vi "Refresh Database Port Compare.vi"(8 "error in":errorcluster, 10 "CAN Cluster":T5, 11 "Port Ref":T8 format="%.0x") -> (0 "error out":errorcluster, 2 "Refresh Port":T1)   [LabVIEW 2020, in "Communication Bus Template System Explorer.lvlib" / "Implementation.lvlib"]
uses:
  Implementation.lvlib
  <vilib>/NI VeriStand/Custom Device API/Custom Device Item Ref.ctl
  Types/Database.ctl
  Types/Frame.ctl
  Types/Signal.ctl
  Types/ECU.ctl
  Types/Refresh Port.ctl
  Types/Refresh Frame.ctl
  Types/Refresh Signal.ctl
  <vilib>/NI VeriStand/Custom Device API/Custom Device Channel Type.ctl
  Scripting/Communication Bus Template Scripting.lvlib
  <vilib>/NI VeriStand/Custom Device API/Custom Device API.lvlib
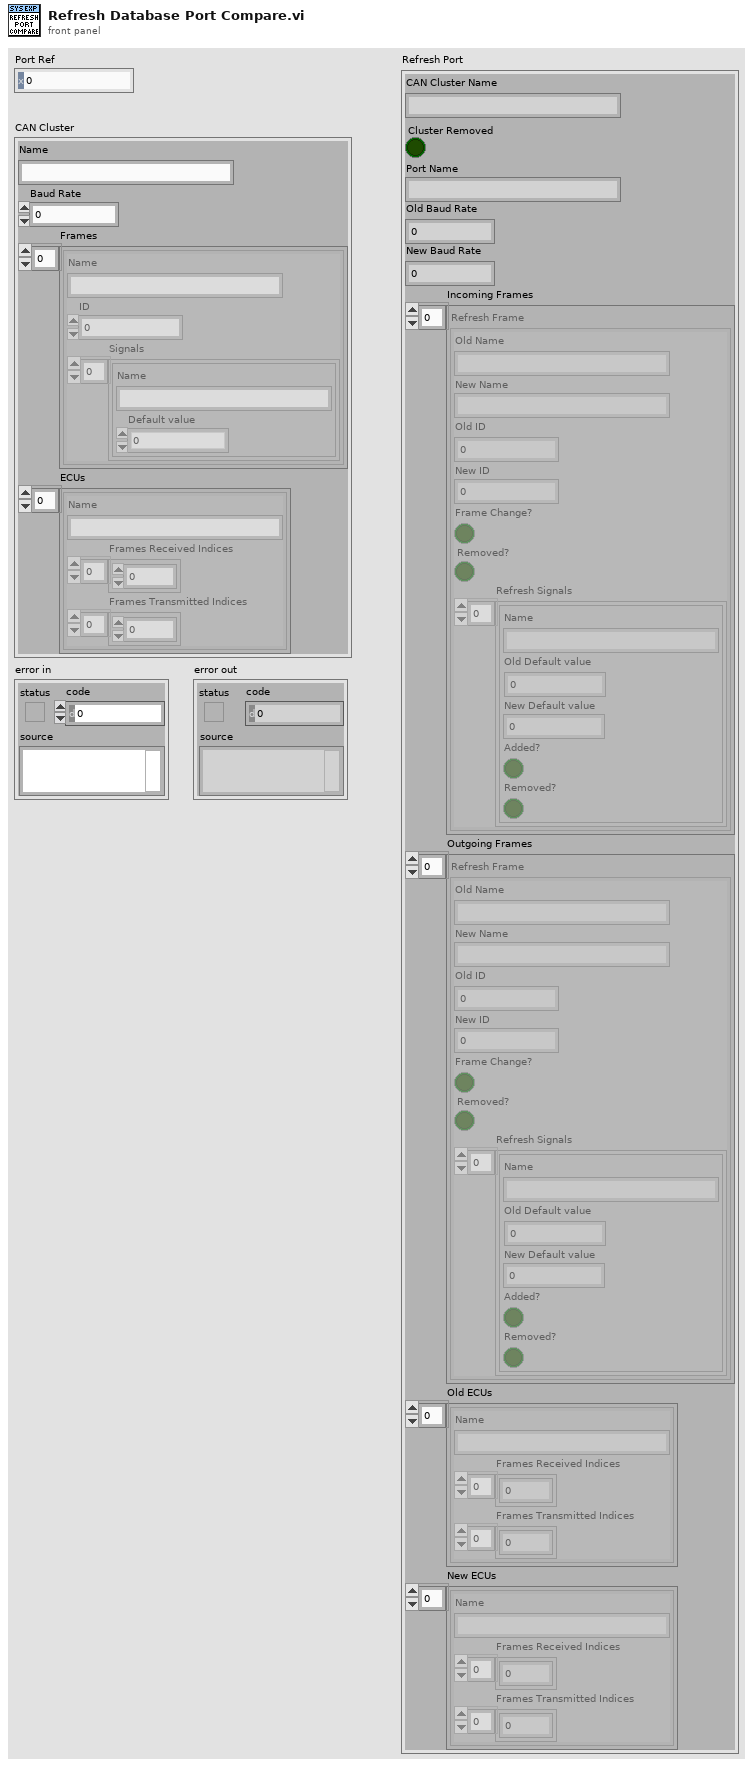
[diagram p1: front panel]
types:
  T1 = typedef "Communication Bus Template System Explorer.lvlib/Implementation.lvlib/Refresh Port.ctl" = cluster{"CAN Cluster Name":string, "Cluster Removed":bool, "Port Name":string, "Old Baud Rate":u64, "New Baud Rate":u64, "Incoming Frames":T2[], "Outgoing Frames":T2[], "Old ECUs":T4[], "New ECUs":T4[]}
  T2 = typedef "Communication Bus Template System Explorer.lvlib/Implementation.lvlib/Refresh Frame.ctl" = cluster{"Old Name":string, "New Name":string, "Old ID":u32, "New ID":u32, "Frame Change?":bool, "Removed?":bool, "Refresh Signals":T3[]}
  T3 = typedef "Communication Bus Template System Explorer.lvlib/Implementation.lvlib/Refresh Signal.ctl" = cluster{"Name":string, "Old Default value":dbl, "New Default value":dbl, "Added?":bool, "Removed?":bool}
  T4 = typedef "Communication Bus Template System Explorer.lvlib/Implementation.lvlib/ECU.ctl" = cluster{"Name":string, "Frames Received Indices":u32[], "Frames Transmitted Indices":u32[]}
  T5 = typedef "Communication Bus Template System Explorer.lvlib/Implementation.lvlib/Database.ctl" = cluster{"Name":string, "Baud Rate":u64, "Frames":T6[], "ECUs":T4[]}
  T6 = typedef "Communication Bus Template System Explorer.lvlib/Implementation.lvlib/Frame.ctl" = cluster{"Name":string, "ID":u32, "Signals":T7[]}
  T7 = typedef "Communication Bus Template System Explorer.lvlib/Implementation.lvlib/Signal.ctl" = cluster{"Name":string, "Default value":dbl}
  T8 = typedef "Custom Device API.lvlib/Custom Device Item Ref.ctl" = u64
  T9 = typedef "Custom Device API.lvlib/Custom Device Channel Type.ctl" = enum16{"Input", "Output"}
  T10 = typedef "Custom Device API.lvlib/Custom Device Channel.ctl" = cluster{"Type":T9, "Units":string, "Default Value":dbl, "Faultable":bool, "Scalable":bool}
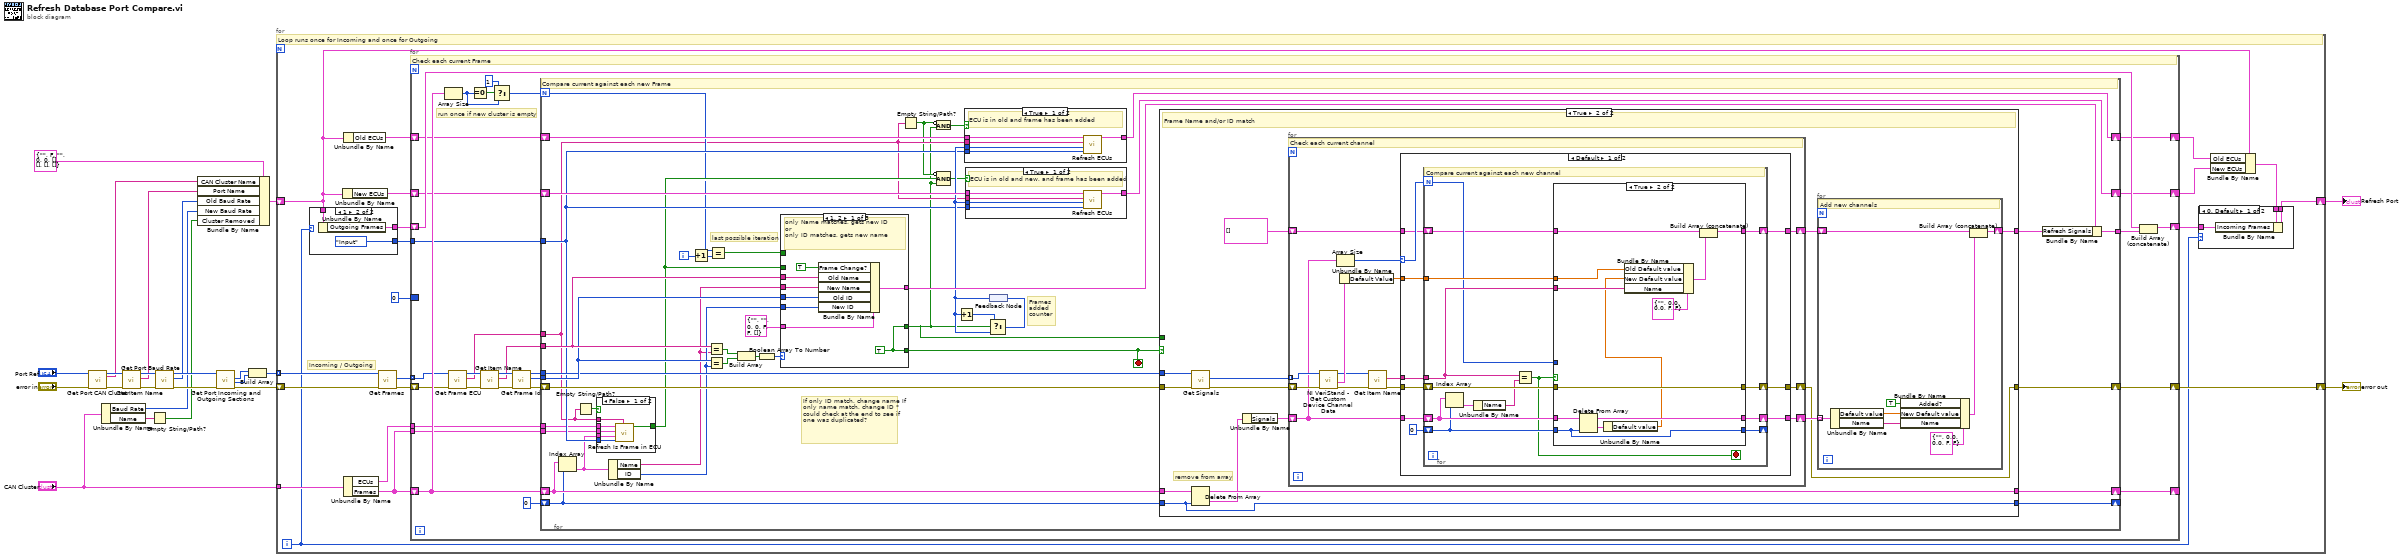
[diagram p0: block diagram]
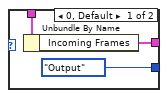
[diagram p2: hidden frame]
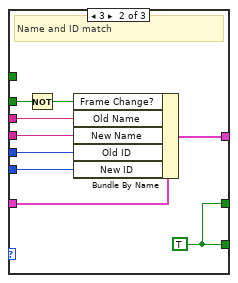
[diagram p6: hidden frame]
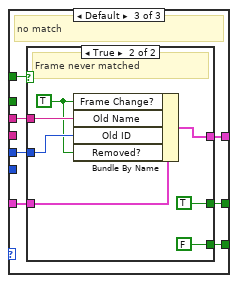
[diagram p7: hidden frame]
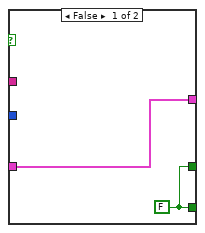
[diagram p8: hidden frame]
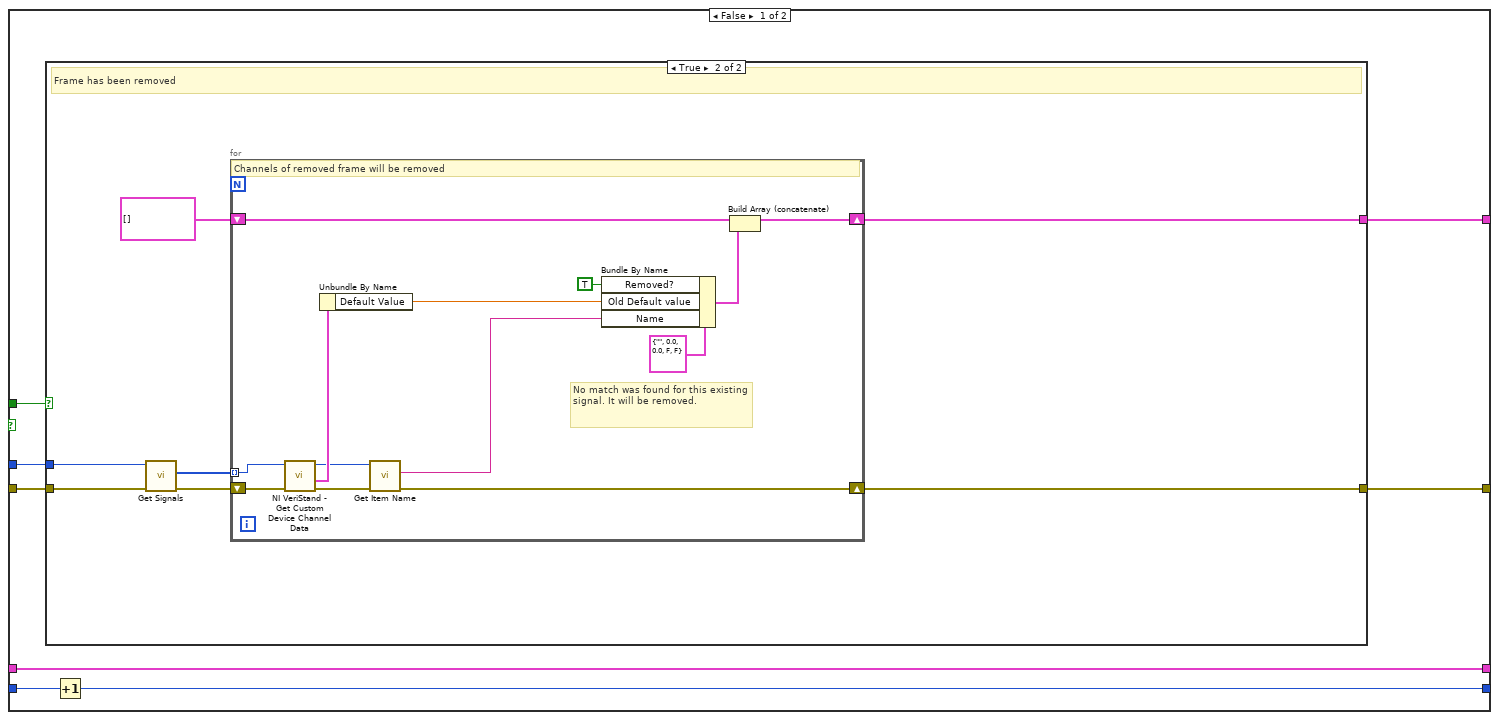
[diagram p9: hidden frame]
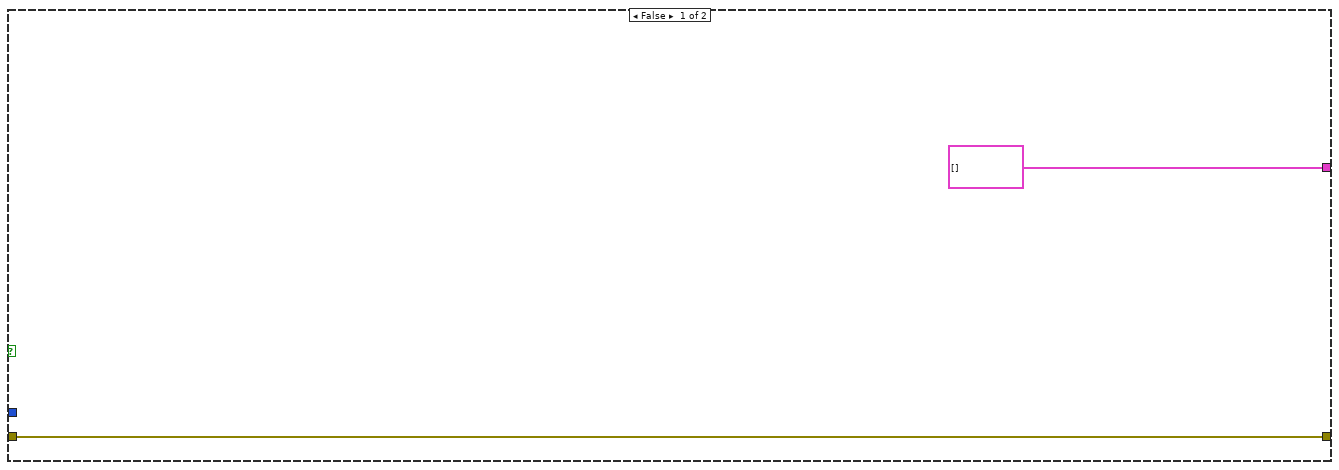
[diagram p10: hidden frame]
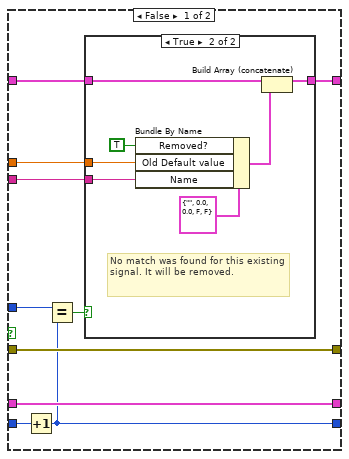
[diagram p11: hidden frame]
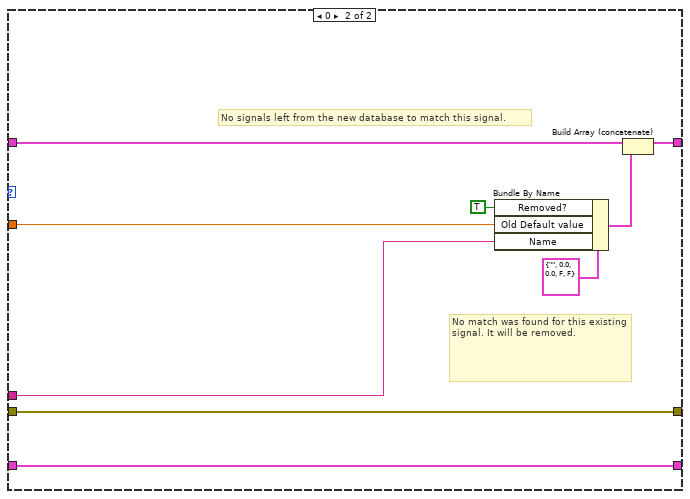
[diagram p13: hidden frame]
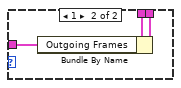
[diagram p14: hidden frame]
diagram:
  n1 = call "Get Port CAN Cluster.vi"("error in"="error in", "Port Ref"="Port Ref") -> ("error out"=w4:errorcluster, "CAN Cluster"=w3:string, "Port Ref out"=w6:T8)  [unwired: 7 in]
  n2 = Unbundle By Name("CAN Cluster") -> ("Baud Rate"=w10:u64, "Name"=w2:string)
  n3 = call "Get Item Name.vi"("error in"=w4, "Item Ref"=w6) -> ("error out"=w15:errorcluster, "Name"=w12:string, "Item Ref out"=w14:T8)  [unwired: 7 in]
  n4 = Empty String/Path?(string/path=w2) -> (empty?=w1:bool)
  n5 = call "Get Port Baud Rate.vi"("error in"=w15, "Port Ref"=w14) -> ("error out"=w22:errorcluster, "Baud Rate"=w11:u32, "Port Ref out"=w23:T8)  [unwired: 7 in]
  n6 = Bundle By Name(cluster=T1 {"CAN Cluster Name"="", "Cluster Removed"=FALSE, "Port Name"="", "Old Baud Rate"=0, "New Baud Rate"=0, "Incoming Frames"=[], "Outgoing Frames"=[], "Old ECUs"=[], "New ECUs"=[]} ("Refresh Port"), "CAN Cluster Name"=w3, "Port Name"=w12, "Old Baud Rate"=w11, "New Baud Rate"=w10, "Cluster Removed"=w1) -> (w9:T1)
  n7 = call "Get Port Incoming and Outgoing Sections.vi"("error in"=w22, "Port Ref"=w23) -> ("error out"=w21:errorcluster, "Outgoing"=w19:T8, "Incoming"=w20:T8)  [unwired: 6 in, 1 out]
  n8 = Build Array(w20, w19) -> (w18:T8[])
  n9 = for {
    shift-right: [w39] -> w16
    shift-left: w21 -> [w43]
    tunnel: w18 -> [w42] mode=indexing
    tunnel: "CAN Cluster" -> [w41]
    shift-right: [w31] -> w8
    shift-left: w9 -> [w30]
    i -> [w35]
    # "Incoming / Outgoing"
    # "Loop runs once for Incoming and once for Outgoing"
    n10 = case shown="1" w35 {
      tunnel: [w45 w49] -> w37
      tunnel: w30 -> [w46 w48]
      tunnel: [Custom_Device_Channel_Type."Output" ("Type (Input)") Custom_Device_Channel_Type."Input" ("Type (Input)")] -> w33
      frame 0, Default {
        n11 = Unbundle By Name(w46) -> ("Incoming Frames"=w45:T2[])
      }
      frame 1 {
        n12 = Unbundle By Name(w48) -> ("Outgoing Frames"=w49:T2[])
      }
    }
    n13 = Unbundle By Name(w30) -> ("New ECUs"=w34:T4[])
    n14 = Unbundle By Name(w41) -> ("ECUs"=w25:T4[], "Frames"=w24:T6[])
    n15 = Unbundle By Name(w30) -> ("Old ECUs"=w32:T4[])
    n16 = call "Get Frames.vi"("error in"=w43, "Incoming/Outgoing in"=w42) -> ("error out"=w40:errorcluster, "Frames"=w38:T8[])  [unwired: 7 in, 1 out]
    n17 = for {
      shift-right: [w70] -> w39
      shift-left: w40 -> [w63]
      tunnel: w38 -> [w64] mode=indexing
      shift-right: [w69] -> _
      shift-left: w24 -> [w73]
      shift-right: [w68] -> w36
      shift-left: w37 -> [w66]
      shift-right: [w57] -> w27
      shift-left: w34 -> [w60]
      tunnel: w33 -> [w59]
      shift-right: [w56] -> w28
      shift-left: w32 -> [w58]
      border: u32 0 ("Frame Index") -> [_]
      tunnel: w25 -> [w55]
      tunnel: w24 -> [w54]
      # "run once if new cluster is empty"
      # "Check each current Frame"
      n18 = Array Size(array=w73) -> (size(s)=w52:i32)
      n19 = call "Get Frame ECU.vi"("error in"=w63, "Frame Ref"=w64) -> ("error out"=w62:errorcluster, "ECU Name"=w61:string, "Frame Ref out"=w65:T8)  [unwired: 7 in]
      n20 = Equal To 0?(x=w52) -> (x = 0?=w53:bool)
      n21 = call "Get Item Name.vi"("error in"=w62, "Item Ref"=w65) -> ("error out"=w78:errorcluster, "Name"=w74:string, "Item Ref out"=w77:T8)  [unwired: 7 in]
      n22 = Select(t=1, s=w53, f=w52) -> (s? t:f=w50:i32)
      n23 = call "Get Frame Id.vi"("error in"=w78, "Frame Ref"=w77) -> ("error out"=w76:errorcluster, "ID"=w75:u32, "Frame Ref out"=w72:T8)  [unwired: 7 in]
      n24 = for {
        N: w50 -> [w84]
        shift-right: [w112] -> w70
        shift-left: w76 -> [w116]
        shift-right: [w117] -> w69
        shift-left: w73 -> [w118]
        tunnel: w75 -> [w119]
        tunnel: w74 -> [w120]
        tunnel: w72 -> [w115]
        shift-right: [w113] -> _
        shift-left: 0 -> [w114]
        tunnel: [w103] -> w67
        tunnel: w61 -> [w81]
        shift-right: [w96] -> w56
        shift-left: w58 -> [w101]
        shift-right: [w97] -> w57
        shift-left: w60 -> [w98]
        tunnel: w59 -> [w91]
        tunnel: w55 -> [w89]
        tunnel: w54 -> [w88]
        i -> [w86]
        stop <- w92 stop-if-true
        # "last possible iteration"
        # "Frames added counter"
        # "If only ID match, change name If only name match, change ID * could check at the end to see if one was duplicated?"
        # "Compare current against each new Frame"
        n25 = Index Array(array=w118, index=w114) -> (element=w90:T6)
        n26 = Empty String/Path?(string/path=w81) -> (empty?=w82:bool)
        n27 = case shown="False" w82 {
          selector: w82 -> [_ w127]
          tunnel: w91 -> [w126 _]
          tunnel: w90 -> [w125 _]
          tunnel: w89 -> [w124 _]
          tunnel: w88 -> [w123 _]
          tunnel: [w122 w127] -> w87
          tunnel: w81 -> [w121 _]
          frame False {
            n28 = call "Refresh Is Frame in ECU.vi"("ECU Name"=w121, "Type (Input)"=w126, "Frame"=w125, "Frames"=w123, "ECUs"=w124) -> ("Found?"=w122:bool)  [unwired: 6 in]
          }
          frame True {
          }
        }
        n29 = Unbundle By Name(w90) -> ("Name"=w107:string, "ID"=w108:u32)
        n30 = Increment(x=w86) -> (x+1=w85:i32)
        n31 = Equal?(x=w120, y=w107) -> (x = y?=w111:bool)
        n32 = Equal?(x=w119, y=w108) -> (x = y?=w110:bool)
        n33 = Equal?(x=w84, y=w85) -> (x = y?=w83:bool)
        n34 = Build Array(w111, w110) -> (w109:bool[])
        n35 = Boolean Array To Number(Boolean array=w109) -> (number=w106:u32)
        n36 = case shown="1, 2" w106 {
          tunnel: w120 -> [w145 w153 w161]
          tunnel: w119 -> [w147 w155 w160]
          tunnel: [w140 w148 w163] -> w92
          tunnel: w108 -> [w142 w156 _]
          tunnel: w107 -> [w146 w154 _]
          tunnel: [w143 w152 w158] -> w105
          tunnel: T2 {"Old Name"="", "New Name"="", "Old ID"=0, "New ID"=0, "Frame Change?"=FALSE, "Removed?"=FALSE, "Refresh Signals"=[]} ("Refresh Frame") -> [w141 w151 w159]
          tunnel: w87 -> [_ w150 _]
          tunnel: w83 -> [_ _ w162]
          tunnel: [w140 w148 w157] -> w79
          frame 1, 2 {
            w140 = TRUE
            # "only Name matches, gets new ID\nor\nonly ID matches, gets new name"
            n37 = Bundle By Name(cluster=w141, "Frame Change?"=TRUE ("ID or Name Change?"), "Old Name"=w145, "New Name"=w146, "Old ID"=w147, "New ID"=w142) -> (w143:T2)
          }
          frame 3 {
            w148 = TRUE
            # "Name and ID match"
            n38 = Not(x=w150) -> (.not. x?=w149:bool)
            n39 = Bundle By Name(cluster=w151, "Frame Change?"=w149, "Old Name"=w153, "New Name"=w154, "Old ID"=w155, "New ID"=w156) -> (w152:T2)
          }
          frame Default {
            # "no match"
            n40 = case shown="True" w162 {
              tunnel: [w164 FALSE] -> w163
              tunnel: w161 -> [_ w171]
              tunnel: w160 -> [_ w170]
              tunnel: w159 -> [w165 w169]
              tunnel: [w165 w168] -> w158
              tunnel: [w164 TRUE] -> w157
              frame False {
                w164 = FALSE
              }
              frame True {
                w166 = TRUE ("ID or Name Change?")
                # "Frame never matched"
                n41 = Bundle By Name(cluster=w169, "Frame Change?"=w166, "Old Name"=w171, "Old ID"=w170, "Removed?"=w166) -> (w168:T2)
              }
            }
          }
        }
        n42 = Empty String/Path?(string/path=w81) -> (empty?=w80:bool)
        n43 = Compound Arithmetic op=AND(invert w80, w79) -> (w94:bool)
        n44 = Compound Arithmetic op=AND(invert w80, w87, w79) -> (w93:bool)
        n45 = feedback #1() -> (w95:u32)
        n46 = Increment(x=w95) -> (x+1=w100:u32)
        n47 = case shown="True" w94 {
          tunnel: w91 -> [w138 _]
          tunnel: w81 -> [w134 _]
          tunnel: w101 -> [w137 w139]
          tunnel: w95 -> [w136 _]
          tunnel: [w135 w139] -> w96
          frame True {
            # "ECU is in old and frame has been added"
            n48 = call "Refresh ECUs.vi"("Type (Input)"=w138, "Frame Index"=w136, "ECU Name"=w134, "ECUs"=w137) -> ("ECUs out"=w135:T4[])  [unwired: 7 in]
          }
          frame False {
          }
        }
        n49 = case shown="True" w93 {
          tunnel: w91 -> [w132 _]
          tunnel: w81 -> [w128 _]
          tunnel: w98 -> [w131 w133]
          tunnel: w95 -> [w130 _]
          tunnel: [w129 w133] -> w97
          frame True {
            # "ECU is in old and new, and frame has been added"
            n50 = call "Refresh ECUs.vi"("Type (Input)"=w132, "Frame Index"=w130, "ECU Name"=w128, "ECUs"=w131) -> ("ECUs out"=w129:T4[])  [unwired: 7 in]
          }
          frame False {
          }
        }
        n51 = Select(t=w100, s=w79, f=w95) -> (s? t:f=w99:u32)
        n52 = feedback-in #1(w99) -> ()
        n53 = case shown="True" w92 {
          tunnel: w118 -> [w180 w216]
          tunnel: w114 -> [w179 w203]
          tunnel: [w180 w215] -> w117
          tunnel: w116 -> [w174 w214]
          tunnel: w115 -> [w175 w213]
          tunnel: [w178 w203] -> w113
          tunnel: [w173 w204] -> w112
          tunnel: [w177 w205] -> w104
          tunnel: w79 -> [w176 _]
          frame False {
            n54 = case shown="True" w176 {
              tunnel: [T3[] [] ("Refresh Signals") w184] -> w177
              tunnel: w175 -> [_ w186]
              tunnel: w174 -> [w181 w185]
              tunnel: [w181 w183] -> w173
              frame False {
              }
              frame True {
                # "Frame has been removed"
                n55 = call "Get Signals.vi"("error in"=w185, "Frame in"=w186) -> ("error out"=w189:errorcluster, "Signals"=w188:T8[])  [unwired: 7 in, 1 out]
                n56 = for {
                  tunnel: w188 -> [w201] mode=indexing
                  shift-right: [w195] -> w183
                  shift-left: w189 -> [w202]
                  shift-right: [w193] -> w184
                  shift-left: T3[] [] ("Refresh Signals") -> [w194]
                  # "No match was found for this existing signal. It will be removed."
                  # "Channels of removed frame will be removed"
                  n57 = call <vilib>:"NI VeriStand - Get Custom Device Channel Data.vi"("error in (no error)"=w202, "Channel Ref in"=w201) -> ("error out"=w198:errorcluster, "Channel"=w200:T10, "Channel Ref out"=w199:T8)  [unwired: 4 in, 3 out]
                  n58 = Unbundle By Name(w200) -> ("Default Value"=w196:dbl)
                  n59 = call "Get Item Name.vi"("error in"=w198, "Item Ref"=w199) -> ("error out"=w195:errorcluster, "Name"=w197:string)  [unwired: 7 in, 1 out]
                  n60 = Bundle By Name(cluster=T3 {"Name"="", "Old Default value"=0.0, "New Default value"=0.0, "Added?"=FALSE, "Removed?"=FALSE} ("Refresh Signal"), "Removed?"=TRUE, "Old Default value"=w196, "Name"=w197) -> (w190:T3)
                  n61 = Build Array (concatenate)(w194, w190) -> (w193:T3[])
                }
              }
            }
            n62 = Increment(x=w179) -> (x+1=w178:i32)
          }
          frame True {
            # "remove from array"
            # "Frame Name and/or ID match"
            n63 = call "Get Signals.vi"("error in"=w214, "Frame in"=w213) -> ("error out"=w212:errorcluster, "Signals"=w211:T8[])  [unwired: 7 in, 1 out]
            n64 = Delete From Array(array=w216, index=w203) -> (deleted portion=w210:T6, array with subset deleted=w215:T6[])  [unwired: 1 in]
            n65 = Unbundle By Name(w210) -> ("Signals"=w209:T7[])
            n66 = for {
              tunnel: w211 -> [w229] mode=indexing
              shift-right: [w220] -> w208
              shift-left: w209 -> [w223]
              shift-right: [w221] -> w204
              shift-left: w212 -> [w230]
              shift-right: [w217] -> w206
              shift-left: T3[] [] ("Refresh Signals") -> [w218]
              # "Check each current channel"
              n67 = call <vilib>:"NI VeriStand - Get Custom Device Channel Data.vi"("error in (no error)"=w230, "Channel Ref in"=w229) -> ("error out"=w226:errorcluster, "Channel"=w228:T10, "Channel Ref out"=w227:T8)  [unwired: 4 in, 3 out]
              n68 = Array Size(array=w223) -> (size(s)=w219:i32)
              n69 = Unbundle By Name(w228) -> ("Default Value"=w222:dbl)
              n70 = call "Get Item Name.vi"("error in"=w226, "Item Ref"=w227) -> ("error out"=w225:errorcluster, "Name"=w224:string)  [unwired: 7 in, 1 out]
              n71 = case shown="Default" w219 {
                selector: w219 -> [w233 _]
                tunnel: w225 -> [w240 w293]
                tunnel: w224 -> [w239 w287]
                tunnel: w223 -> [w237 w292]
                tunnel: w222 -> [w236 w286]
                tunnel: [w235 w293] -> w221
                tunnel: [w234 w292] -> w220
                tunnel: w218 -> [w232 w288]
                tunnel: [w231 w285] -> w217
                frame Default {
                  n72 = for {
                    N: w233 -> [w243]
                    shift-right: [w248] -> w234
                    shift-left: w237 -> [w251]
                    shift-right: [w244] -> w235
                    shift-left: w240 -> [w254]
                    tunnel: w239 -> [w247]
                    shift-right: [w249] -> _
                    shift-left: 0 -> [w250]
                    tunnel: w236 -> [w245]
                    shift-right: [w241] -> w231
                    shift-left: w232 -> [w242]
                    stop <- w246 stop-if-true
                    # "Compare current against each new channel"
                    n73 = Index Array(array=w251, index=w250) -> (element=w253:T7)
                    n74 = Unbundle By Name(w253) -> ("Name"=w252:string)
                    n75 = Equal?(x=w247, y=w252) -> (x = y?=w246:bool)
                    n76 = case shown="True" w246 {
                      tunnel: w254 -> [w261 w280]
                      tunnel: w251 -> [w264 w284]
                      tunnel: w250 -> [w257 w283]
                      tunnel: [w258 w283] -> w249
                      tunnel: [w264 w282] -> w248
                      tunnel: w247 -> [w259 w275]
                      tunnel: w245 -> [w262 w273]
                      tunnel: w243 -> [w260 _]
                      tunnel: [w261 w280] -> w244
                      tunnel: w242 -> [w256 w276]
                      tunnel: [w255 w277] -> w241
                      frame False {
                        n77 = Increment(x=w257) -> (x+1=w258:i32)
                        n78 = Equal?(x=w260, y=w258) -> (x = y?=w263:bool)
                        n79 = case shown="True" w263 {
                          tunnel: w259 -> [_ w269]
                          tunnel: w262 -> [_ w268]
                          tunnel: w256 -> [w265 w272]
                          tunnel: [w265 w271] -> w255
                          frame False {
                          }
                          frame True {
                            # "No match was found for this existing signal. It will be removed."
                            n80 = Bundle By Name(cluster=T3 {"Name"="", "Old Default value"=0.0, "New Default value"=0.0, "Added?"=FALSE, "Removed?"=FALSE} ("Refresh Signal"), "Removed?"=TRUE, "Old Default value"=w268, "Name"=w269) -> (w266:T3)
                            n81 = Build Array (concatenate)(w272, w266) -> (w271:T3[])
                          }
                        }
                      }
                      frame True {
                        n82 = Delete From Array(array=w284, index=w283) -> (deleted portion=w281:T7, array with subset deleted=w282:T7[])  [unwired: 1 in]
                        n83 = Unbundle By Name(w281) -> ("Default value"=w274:dbl)
                        n84 = Bundle By Name(cluster=T3 {"Name"="", "Old Default value"=0.0, "New Default value"=0.0, "Added?"=FALSE, "Removed?"=FALSE} ("Refresh Signal"), "Old Default value"=w273, "New Default value"=w274, "Name"=w275) -> (w278:T3)
                        n85 = Build Array (concatenate)(w276, w278) -> (w277:T3[])
                      }
                    }
                  }
                }
                frame 0 {
                  # "No signals left from the new database to match this signal."
                  # "No match was found for this existing signal. It will be removed."
                  n86 = Bundle By Name(cluster=T3 {"Name"="", "Old Default value"=0.0, "New Default value"=0.0, "Added?"=FALSE, "Removed?"=FALSE} ("Refresh Signal"), "Removed?"=TRUE, "Old Default value"=w286, "Name"=w287) -> (w289:T3)
                  n87 = Build Array (concatenate)(w288, w289) -> (w285:T3[])
                }
              }
            }
            n88 = for {
              tunnel: w208 -> [w301] mode=indexing
              shift-right: [w297] -> w205
              shift-left: w206 -> [w298]
              # "Add new channels"
              n89 = Unbundle By Name(w301) -> ("Default value"=w295:dbl, "Name"=w296:string)
              n90 = Bundle By Name(cluster=T3 {"Name"="", "Old Default value"=0.0, "New Default value"=0.0, "Added?"=FALSE, "Removed?"=FALSE} ("Refresh Signal"), "Added?"=TRUE, "New Default value"=w295, "Name"=w296) -> (w300:T3)
              n91 = Build Array (concatenate)(w298, w300) -> (w297:T3[])
            }
          }
        }
        n92 = Bundle By Name(cluster=w105, "Refresh Signals"=w104) -> (w103:T2)
      }
      n93 = Build Array (concatenate)(w66, w67) -> (w68:T2[])
    }
    n94 = Bundle By Name(cluster=w30, "Old ECUs"=w28, "New ECUs"=w27) -> (w29:T1)
    n95 = case shown="0, Default" w35 {
      tunnel: w29 -> [w304 w307]
      tunnel: [w303 w306] -> w31
      tunnel: w36 -> [w302 w305]
      frame 0, Default {
        n96 = Bundle By Name(cluster=w304, "Incoming Frames"=w302) -> (w303:T1)
      }
      frame 1 {
        n97 = Bundle By Name(cluster=w307, "Outgoing Frames"=w305) -> (w306:T1)
      }
    }
  }
  "error out" <- w16
  "Refresh Port" <- w8
